vi "tcp_client_Rx_y_Tx_1_5.vi"() -> ()   [LabVIEW 2020]
panel:
  out "Gauge":dbl(knob) scale=0.0..1023.0
  out "Numeric":dbl
  in  "COMANDO":string
  in  "ENVIAR":bool
  in  "OFF":bool
  in  "ON":bool
  out "Waveform Chart":dbl(graph)
  in  "stop":bool
  out "data out":string
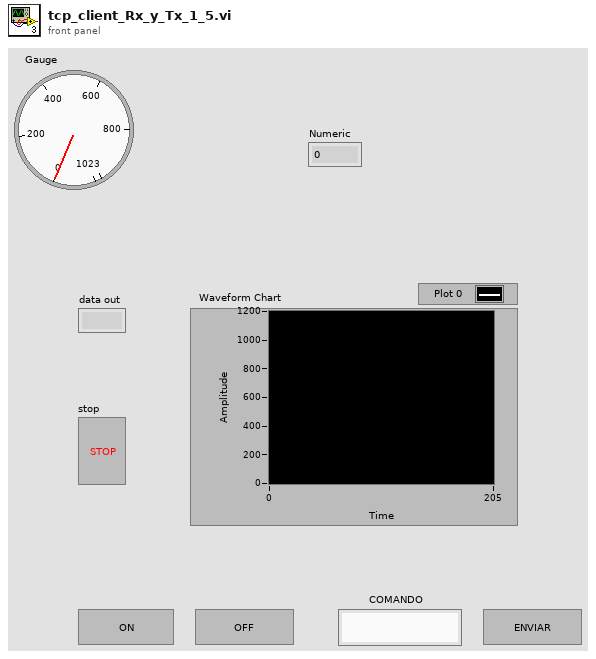
[diagram p1: front panel]
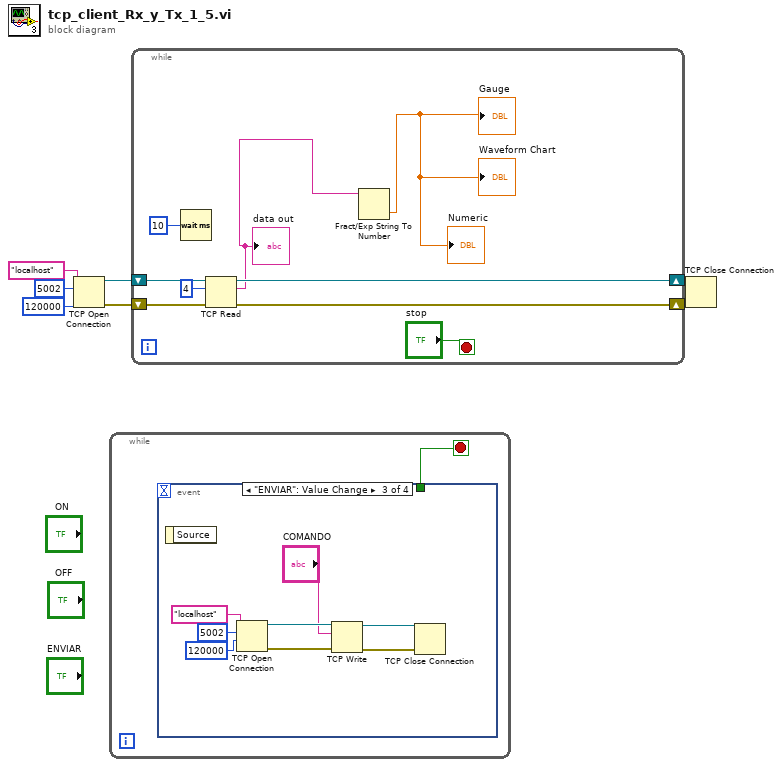
[diagram p0: block diagram]
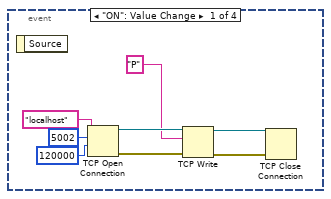
[diagram p2: hidden frame]
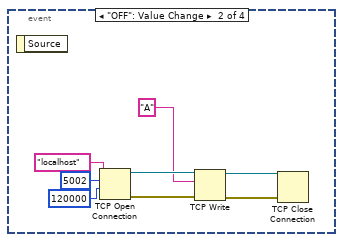
[diagram p3: hidden frame]
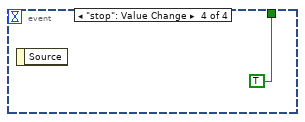
[diagram p4: hidden frame]
diagram:
  n1 = TCP Open Connection(address="localhost", remote port or service name=u16 5002, timeout ms (60000)=120000) -> (connection ID=w2:refnum<k5>, error out=w1:errorcluster)  [unwired: 2 in]
  n2 = while {
    stop <- w8 stop-if-true
    n3 = event shown="[2] \"ENVIAR\": Value Change" {
      selector: _ -> [_ _ _ _]
      dyn-events: _ -> [_ _ _ _]
      timeout: _ -> [_ _ _ _]
      tunnel: [_ _ _ TRUE] -> w8
      event "ON": Value Change {
        n4 = event-data() -> ()  [unwired: 1 in, 1 out]
        n5 = TCP Open Connection(address="localhost", remote port or service name=u16 5002, timeout ms (60000)=120000) -> (connection ID=w16:refnum<k5>, error out=w15:errorcluster)  [unwired: 2 in]
        n6 = TCP Write(connection ID=w16, data in="P", error in (no error)=w15) -> (connection ID out=w14:refnum<k5>, error out=w13:errorcluster)  [unwired: 1 in, 1 out]
        n7 = TCP Close Connection(connection ID=w14, error in (no error)=w13) -> ()  [unwired: 1 in, 2 out]
      }
      event "OFF": Value Change {
        n8 = event-data() -> ()  [unwired: 1 in, 1 out]
        n9 = TCP Open Connection(address="localhost", remote port or service name=u16 5002, timeout ms (60000)=120000) -> (connection ID=w24:refnum<k5>, error out=w23:errorcluster)  [unwired: 2 in]
        n10 = TCP Write(connection ID=w24, data in="A", error in (no error)=w23) -> (connection ID out=w22:refnum<k5>, error out=w21:errorcluster)  [unwired: 1 in, 1 out]
        n11 = TCP Close Connection(connection ID=w22, error in (no error)=w21) -> ()  [unwired: 1 in, 2 out]
      }
      event "ENVIAR": Value Change {
        n12 = event-data() -> ()  [unwired: 1 in, 1 out]
        n13 = TCP Open Connection(address="localhost", remote port or service name=u16 5002, timeout ms (60000)=120000) -> (connection ID=w29:refnum<k5>, error out=w30:errorcluster)  [unwired: 2 in]
        n14 = TCP Write(connection ID=w29, data in="COMANDO", error in (no error)=w30) -> (connection ID out=w31:refnum<k5>, error out=w32:errorcluster)  [unwired: 1 in, 1 out]
        n15 = TCP Close Connection(connection ID=w31, error in (no error)=w32) -> ()  [unwired: 1 in, 2 out]
      }
      event "stop": Value Change {
        n16 = event-data() -> ()  [unwired: 1 in, 1 out]
      }
    }
  }
  n17 = while {
    shift-right: [w41] -> w7
    shift-left: w2 -> [w42]
    shift-right: [w39] -> w6
    shift-left: w1 -> [w40]
    stop <- "stop" stop-if-true
    n18 = Wait (ms)(milliseconds to wait=u32 10) -> ()  [unwired: 1 out]
    n19 = TCP Read(connection ID=w42, bytes to read=4, error in (no error)=w40) -> (connection ID out=w41:refnum<k5>, data out=w35:string, error out=w39:errorcluster)  [unwired: 2 in]
    "data out" <- w35
    n20 = Fract/Exp String To Number(string=w35) -> (number=→"Numeric" →"Waveform Chart" →"Gauge":dbl)  [unwired: 3 in, 1 out]
  }
  n21 = TCP Close Connection(connection ID=w7, error in (no error)=w6) -> ()  [unwired: 1 in, 2 out]
